vi "Post Build Package Mods -- Wrapper.vi"(8 "error in (no error)":errorcluster, 9 "Built package path":path, 11 "Project Root":path) -> (0 "error out":errorcluster)   [LabVIEW 2013]
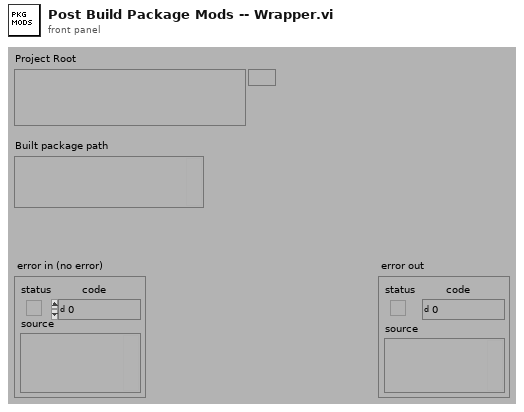
[diagram p1: front panel]
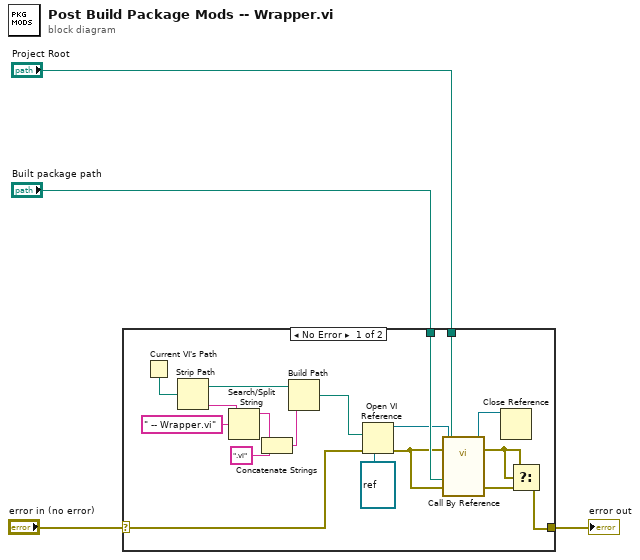
[diagram p0: block diagram]
diagram:
  n1 = case shown="No Error" "error in (no error)" {
    selector: "error in (no error)" -> [w14 w23]
    tunnel: [w20 w23] -> w3
    tunnel: "Built package path" -> [w22 _]
    tunnel: "Project Root" -> [w13 _]
    frame No Error {
      n2 = Current VI's Path() -> (path=w12:path)
      n3 = Strip Path(path=w12) -> (stripped path=w11:path, name=w9:string)
      n4 = Search/Split String(string=w9, search string/char (-)=" -- Wrapper.vi") -> (substring before match=w7:string)  [unwired: 1 in, 2 out]
      n5 = Concatenate Strings(w7, ".vi" ("string")) -> (w5:string)
      n6 = Build Path(base path=w11, name or relative path=w5) -> (appended path=w10:path)
      n7 = Open VI Reference(type specifier VI Refnum (for type only)=refnum<vi> refnum, vi path=w10, error in (no error)=w14) -> (vi reference=w17:refnum<vi>, error out=w15:errorcluster)  [unwired: 3 in]
      n8 = call-by-ref "?"(reference=w17, error in=w15, "error in (no error)"=w15, "Built package path"=w22, "Project Root"=w13) -> (reference out=w18:refnum<vi>, error out=w19:errorcluster, 0:"error out"=w21:errorcluster)  [unwired: 8 in]
      n9 = Close Reference(reference=w18) -> ()  [unwired: 1 in, 1 out]
      n10 = Select(t=w19, s=w19, f=w21) -> (s? t:f=w20:errorcluster)
    }
    frame Error {
    }
  }
  "error out" <- w3
